vi "LVFunction_Imop_Compute_LegendrePupil.vi"(0 "Pupil.lvclass":refnum<class "Pupil.lvclass">, 5 "SquarePupilDetectionParams":T2, 7 "center in":T1, 9 "size in":T1, 11 "error in":errorcluster) -> (4 "Pupil.lvclass":refnum<class "Pupil.lvclass">, 8 "center out":T1, 10 "size out":T1, 15 "error out":errorcluster)   [LabVIEW 2018]
doc: "Compute the geometric parameters of the Legendre pupil from a pupil input.\n\n<B>PupilIn</B> : pupil object.\n<B>PupilOut</B> : pupil object.\n<B>center</B> : center coordinates. Values are expressed in subpupils.\n<B>size</B> : dimensions (width, height) of the square pupil detected. Values are expressed in number of subpupils."
uses:
  Classes/Pupil/Pupil.lvclass
  Controls/Point2Df.ctl
  Controls/SquarePupilDetectionParams.ctl
  Controls/PupilDetectionOption.ctl
  Classes/Pupil/LVClass_Pupil Read Pupil.vi
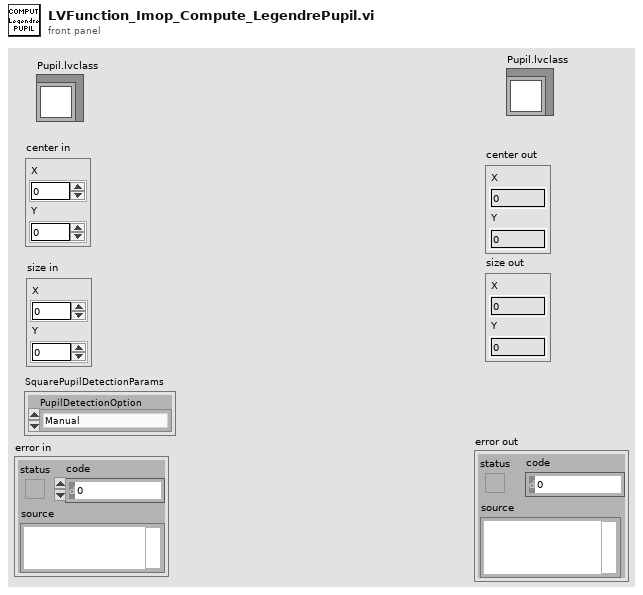
[diagram p1: front panel]
types:
  T1 = typedef "Point2Df.ctl" = cluster{"X":sgl, "Y":sgl}
  T2 = typedef "SquarePupilDetectionParams.ctl" = cluster{"PupilDetectionOption":T3}
  T3 = typedef "PupilDetectionOption.ctl" = enum16{"Manual", "Automatic"}
  T4 = typedef "ClassID.ctl" = i64
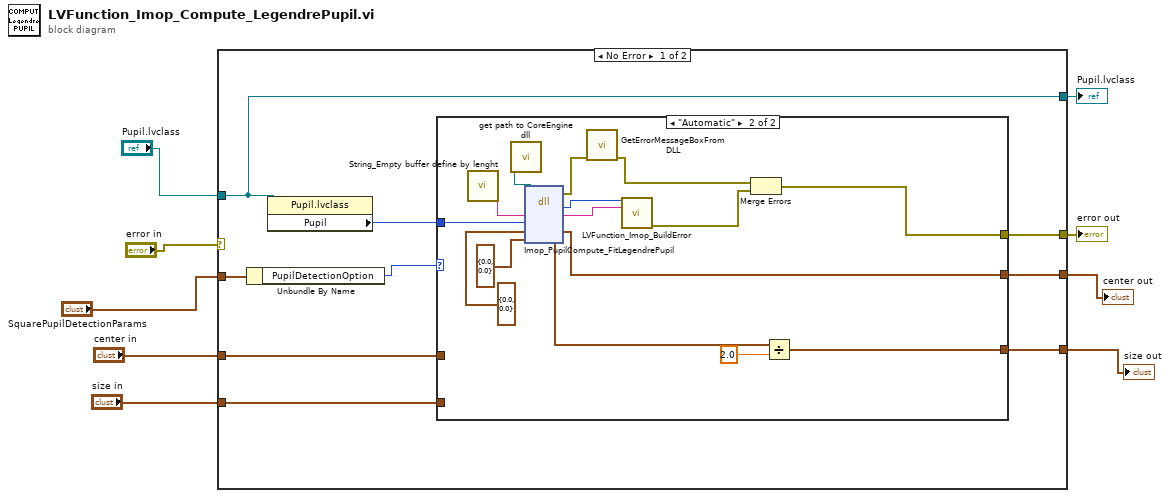
[diagram p0: block diagram]
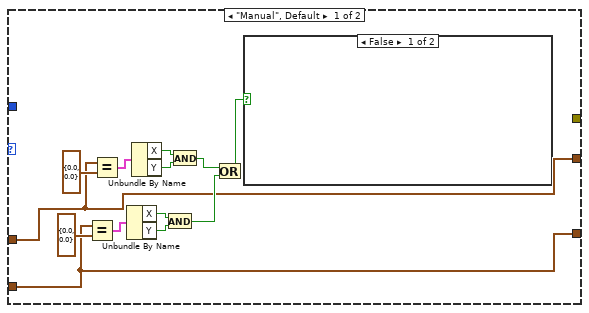
[diagram p2: hidden frame]
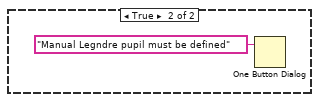
[diagram p3: hidden frame]
diagram:
  n1 = case shown="No Error" "error in" {
    selector: "error in" -> [_ w49]
    tunnel: "Pupil.lvclass" -> [w15 w48]
    tunnel: "SquarePupilDetectionParams" -> [w17 _]
    tunnel: [w16 w49] -> w7
    tunnel: [w15 w48] -> w5
    tunnel: "center in" -> [w13 _]
    tunnel: "size in" -> [w12 _]
    tunnel: [w11 _] -> w2
    tunnel: [w10 _] -> w1
    frame No Error {
      n2 = Unbundle By Name(w17) -> ("PupilDetectionOption"=w14:T3)
      n3 = property class="Pupil.lvclass"(reference=w15) -> ("Pupil"=w18:T4)  [unwired: 1 in, 2 out]
      n4 = case shown="\"Automatic\"" w14 {
        tunnel: w18 -> [_ w42]
        tunnel: [_ w36] -> w16
        tunnel: w13 -> [w20 _]
        tunnel: w12 -> [w19 _]
        tunnel: [w20 w39] -> w11
        tunnel: [w19 w33] -> w10
        frame "Manual", Default {
          n5 = Equal?(x=w19, y=T1 {"X"=0.0, "Y"=0.0}) -> (x = y?=w25:cluster{"X":bool, "Y":bool})
          n6 = Equal?(x=w20, y=T1 {"X"=0.0, "Y"=0.0}) -> (x = y?=w28:cluster{"X":bool, "Y":bool})
          n7 = Unbundle By Name(w25) -> ("X"=w24:bool, "Y"=w23:bool)
          n8 = Unbundle By Name(w28) -> ("X"=w29:bool, "Y"=w30:bool)
          n9 = And(x=w24, y=w23) -> (x .and. y?=w22:bool)
          n10 = And(x=w29, y=w30) -> (x .and. y?=w31:bool)
          n11 = Or(x=w31, y=w22) -> (x .or. y?=w21:bool)
          n12 = case shown="False" w21 {
            frame False {
            }
            frame True {
              n13 = One Button Dialog(message="Manual Legndre pupil must be defined") -> ()  [unwired: 1 in, 1 out]
            }
          }
        }
        frame "Automatic" {
          n14 = call "String_Empty buffer define by lenght.vi"() -> ("Empty buffer"=w47:string)  [unwired: 1 in]
          n15 = call "get path to CoreEngine dll.vi"() -> ("path to wavekit library"=w44:path)  [unwired: 14 in, 1 out]
          n16 = dll-call lib="D:/FLE/0.Code/CoreEngine4_Suite/LV2011_interface/DLLs/c_interface_vc100.dll" fn="Imop_PupilCompute_FitLegendrePupil"(path in=w44, "message"=w47, "Pupil"=w42, "center"=T1 {"X"=0.0, "Y"=0.0}, "taille"=T1 {"X"=0.0, "Y"=0.0}) -> (error out=w43:errorcluster, "return type"=w45:i32, "message"=w46:string, "center"=w39:T1, "taille"=w34:T1)  [unwired: 3 in, 1 out]
          n17 = call "GetErrorMessageBoxFromDLL.vi"("error IN"=w43) -> ("error OUT"=w38:errorcluster)  [unwired: 10 in]
          n18 = call "LVFunction_Imop_BuildError.vi"("code"=w45, "String to Prepend to source (\"\")"=w46) -> ("error out"=w37:errorcluster)  [unwired: 13 in]
          n19 = Merge Errors(w38, w37) -> (w36:errorcluster)
          n20 = Divide(x=w34, y=sgl 2.0 ("Y")) -> (x/y=w33:T1)
        }
      }
    }
    frame Error {
    }
  }
  "error out" <- w7
  "Pupil.lvclass" <- w5
  "center out" <- w2
  "size out" <- w1
